vi "ModifyProjectBuildOutput.vi"() -> ()   [LabVIEW 2020]
panel:
  out "Custom Parameters":string[](array[string])
  out "error out":errorcluster
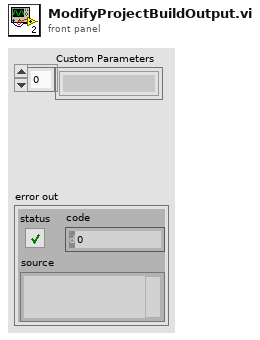
[diagram p1: front panel]
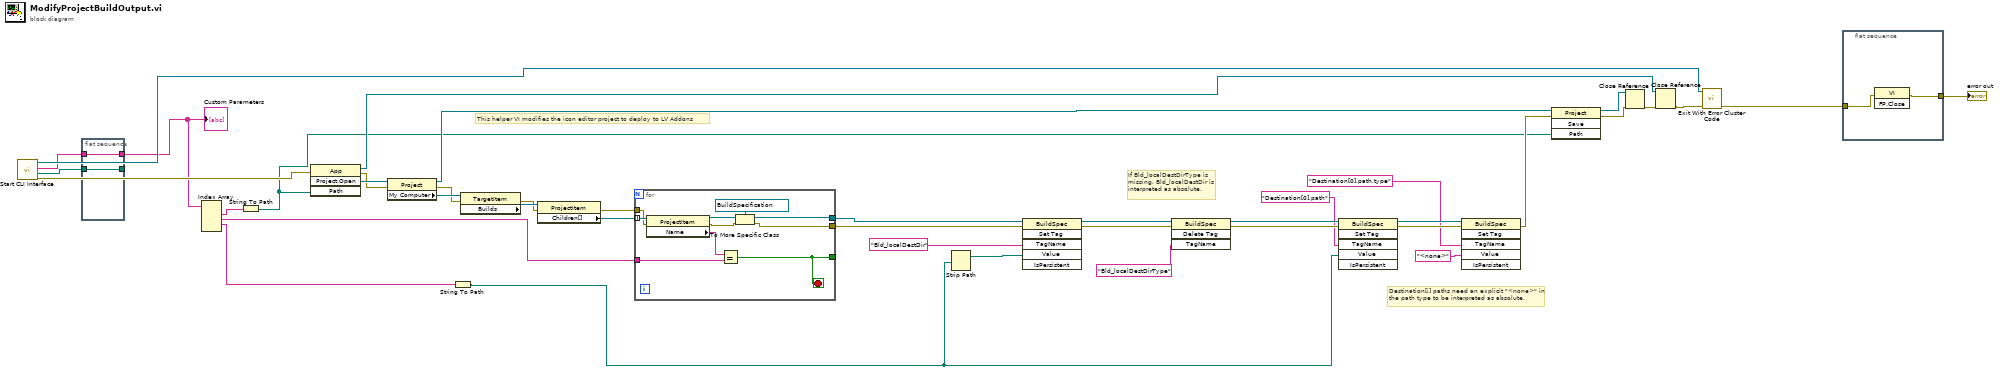
[diagram p0: block diagram]
diagram:
  # "Destination[i] paths need an explicit \"<none>\" in the path type to be interpreted as absolute."
  # "If Bld_localDestDirType is missing, Bld_localDestDir is interpreted as absolute."
  # "This helper VI modifies the icon editor project to deploy to LV Addons"
  n1 = call <vilib>:"Start CLI Interface.vi"() -> ("error out"=w13:errorcluster, "Working Directory"=w8:path, "Custom Parameters"=w7:string[], "CLI out"=w11:refnum<class "CLI.lvclass">)  [unwired: 8 in]
  n2 = flat-sequence {
    tunnel: w8 -> [w43]
    tunnel: [w43] -> _
    tunnel: w7 -> [w42]
    tunnel: [w42] -> w6
    frame #0 {
    }
  }
  n3 = Index Array(array=w6) -> (element #1=w5:string, element #2=w3:string, element #3=w1:string)  [unwired: 4 in, 1 out]
  n4 = String To Path(string=w5) -> (path=w4:path)
  n5 = invoke class="App" method="Project.Open"(error in=w13, "Path"=w4) -> (reference out=w14:refnum<vi>, error out=w21:errorcluster, "Project:Open"=w36:refnum<vi>)  [unwired: 2 in, 1 out]
  n6 = property class="Project"(reference=w36, error in=w21) -> (reference out=w35:refnum<vi>, error out=w20:errorcluster, "My Computer"=w41:refnum<vi>)
  n7 = String To Path(string=w1) -> (path=w2:path)
  n8 = property class="TargetItem"(reference=w41, error in=w20) -> (error out=w19:errorcluster, "Builds"=w39:refnum<vi>)  [unwired: 1 out]
  n9 = property class="ProjectItem"(reference=w39, error in=w19) -> (error out=w18:errorcluster, "Children[]"=w40:refnum<vi>[])  [unwired: 1 out]
  n10 = for {
    tunnel: w40 -> [w53] mode=indexing
    tunnel: [w46] -> w38
    tunnel: w3 -> [w51]
    tunnel: [w50] -> _
    tunnel: [w47] -> w37
    tunnel: w18 -> [w44]
    stop <- w50 stop-if-true
    n11 = property class="ProjectItem"(reference=w53, error in=w44) -> (reference out=w48:refnum<vi>, error out=w49:errorcluster, "Name"=w52:string)
    n12 = Equal?(x=w52, y=w51) -> (x = y?=w50:bool)
    n13 = To More Specific Class(target class=refnum<vi> refnum ("Build Spec"), reference=w48, error in=w49) -> (specific class reference=w46:refnum<vi>, error out=w47:errorcluster)
  }
  n14 = Strip Path(path=w2) -> (stripped path=w22:path)  [unwired: 1 out]
  n15 = invoke class="BuildSpec" method="Set Tag"(reference=w38, error in=w37, "TagName"="Bld_localDestDir" ("Tag Name"), "Value"=w22) -> (reference out=w34:refnum<vi>, error out=w30:errorcluster)  [unwired: 2 in, 4 out]
  n16 = invoke class="BuildSpec" method="Delete Tag"(reference=w34, error in=w30, "TagName"="Bld_localDestDirType" ("Tag Name")) -> (reference out=w33:refnum<vi>, error out=w29:errorcluster)  [unwired: 1 in, 2 out]
  n17 = invoke class="BuildSpec" method="Set Tag"(reference=w33, error in=w29, "TagName"="Destination[0].path" ("format string"), "Value"=w2) -> (reference out=w28:refnum<vi>, error out=w27:errorcluster)  [unwired: 2 in, 4 out]
  n18 = invoke class="BuildSpec" method="Set Tag"(reference=w28, error in=w27, "TagName"="Destination[0].path.type" ("format string"), "Value"="<none>") -> (error out=w23:errorcluster)  [unwired: 2 in, 5 out]
  n19 = invoke class="Project" method="Save"(reference=w35, error in=w23, "Path"=w4) -> (reference out=w16:refnum<vi>, error out=w17:errorcluster)  [unwired: 1 in, 2 out]
  n20 = Close Reference(reference=w16, error in (no error)=w17) -> (error out=w15:errorcluster)
  n21 = Close Reference(reference=w14, error in (no error)=w15) -> (error out=w12:errorcluster)
  n22 = call <vilib>:"Exit With Error Cluster Code.vi"("error in (no error)"=w12, "CLI in"=w11) -> ("error out"=w10:errorcluster)  [unwired: 9 in]
  n23 = flat-sequence {
    tunnel: [w55] -> w9
    tunnel: w10 -> [w54]
    frame #0 {
      n24 = invoke class="VI" method="FP.Close"(error in=w54) -> (error out=w55:errorcluster)  [unwired: 2 in, 2 out]
    }
  }
  "error out" <- w9
  "Custom Parameters" <- w6
